vi "Read Fill Style.vi"(8 "error in (no error)":errorcluster, 11 "Slide.lvclass in":refnum<class "Slide.lvclass">) -> (0 "error out":errorcluster, 2 "FillStyle":i32, 3 "Slide.lvclass out":refnum<class "Slide.lvclass">)   [LabVIEW 2015, in "Slide.lvclass"]
uses:
  Slide.lvclass
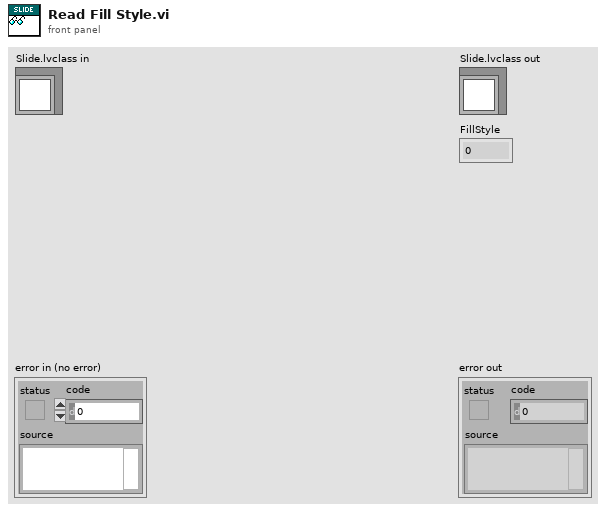
[diagram p1: front panel]
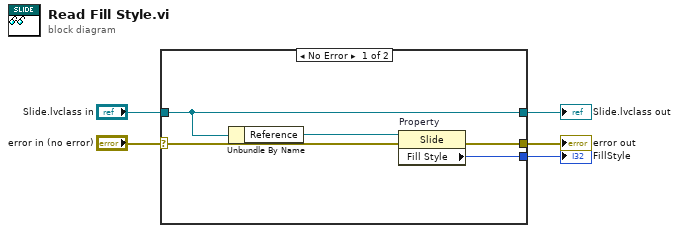
[diagram p0: block diagram]
diagram:
  n1 = case shown="No Error" "error in (no error)" {
    selector: "error in (no error)" -> [w6 w12]
    tunnel: [w9 w12] -> w4
    tunnel: [w8 w11] -> w2
    tunnel: "Slide.lvclass in" -> [w8 w11]
    tunnel: [w10 _] -> w1
    frame No Error {
      n2 = Unbundle By Name(w8) -> ("Reference"=w7:refnum<vi>)
      n3 = property on="Property" class="Slide"(reference=w7, error in=w6) -> (error out=w9:errorcluster, "Fill Style"=w10:i32)  [unwired: 1 out]
    }
    frame Error {
    }
  }
  "error out" <- w4
  "Slide.lvclass out" <- w2
  "FillStyle" <- w1
